vi "PhaseShiftModulation.vi"(0 "PhaseShift":i32, 1 "enable":bool=TRUE, 5 "Period":u32, 7 "Deadband":u8) -> (4 "PrimaryCmds":T1, 6 "SecondaryCmds":T1)   [LabVIEW 2016]
uses:
  BridgeCmds.ctl
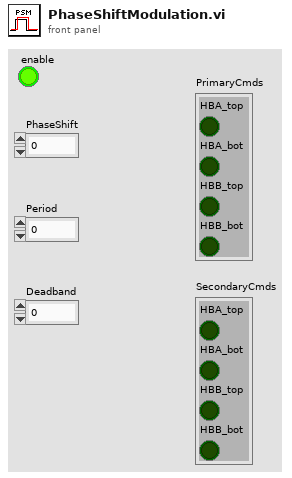
[diagram p1: front panel]
types:
  T1 = typedef "BridgeCmds.ctl" = cluster{"HBA_top":bool, "HBA_bot":bool, "HBB_top":bool, "HBB_bot":bool}
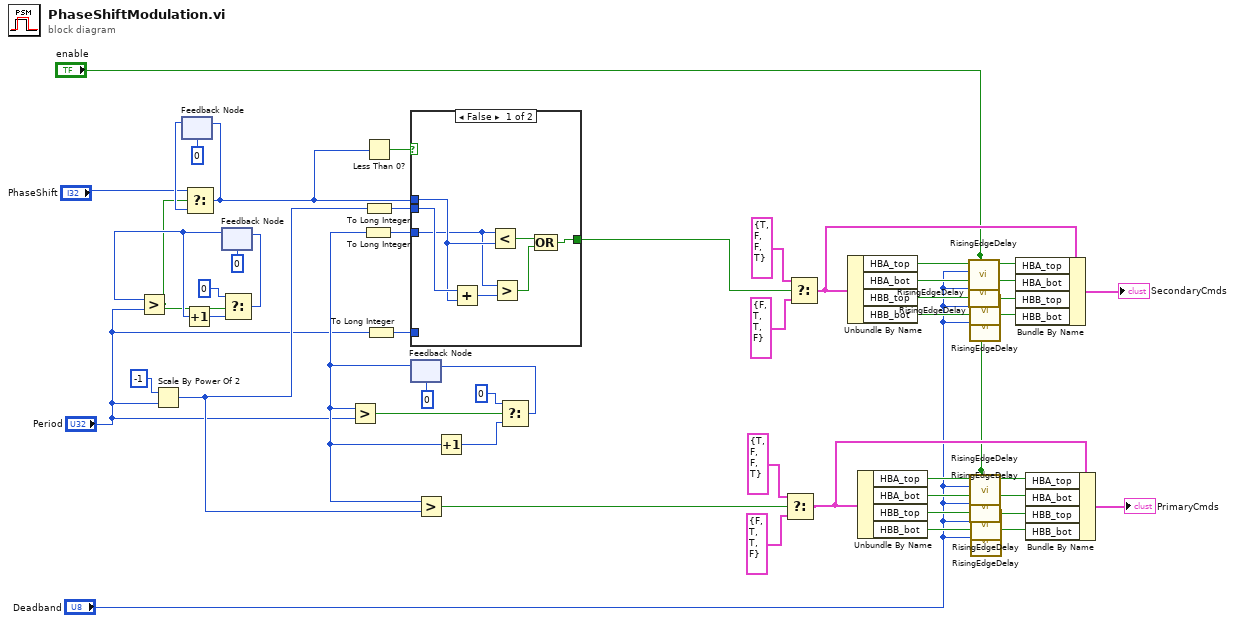
[diagram p0: block diagram]
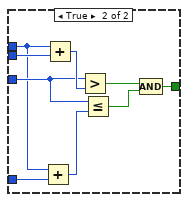
[diagram p2: hidden frame]
diagram:
  n1 = Scale By Power Of 2(n=i16 -1, x="Period") -> (x*2^n=w7:u32)
  n2 = feedback #1(0) -> (w39:i32)
  n3 = feedback #2(u32 0) -> (w41:u32)
  n4 = Greater?(x=w41, y="Period") -> (0:w37:bool)
  n5 = Increment(x=w41) -> (x+1=w43:u32)
  n6 = Select(t="PhaseShift", s=w37, f=w39) -> (s? t:f=w2:i32)
  n7 = feedback-in #1(w2) -> ()
  n8 = Select(t=u32 0, s=w37, f=w43) -> (s? t:f=w42:u32)
  n9 = feedback-in #2(w42) -> ()
  n10 = Less Than 0?(x=w2) -> (x < 0?=w1:bool)
  n11 = To Long Integer(number=w7) -> (32bit integer=w8:i32)
  n12 = To Long Integer(number="Period") -> (32bit integer=w4:i32)
  n13 = feedback #3(u32 0) -> (w6:u32)
  n14 = Greater?(x=w6, y="Period") -> (0:w47:bool)
  n15 = To Long Integer(number=w6) -> (32bit integer=w5:i32)
  n16 = case shown="False" w1 {
    tunnel: [w57 w64] -> w9
    tunnel: w8 -> [w56 w63]
    tunnel: w5 -> [w53 w62]
    tunnel: w4 -> [_ w61]
    tunnel: w2 -> [w55 w59]
    frame False {
      n17 = Add(x=w56, y=w55) -> (x+y=w54:i32)
      n18 = Less?(x=w53, y=w55) -> (x < y?=w58:bool)
      n19 = Greater?(x=w53, y=w54) -> (0:w52:bool)
      n20 = Compound Arithmetic op=OR(w58, w52) -> (w57:bool)
    }
    frame True {
      n21 = Add(x=w59, y=w61) -> (x+y=w60:i32)
      n22 = Add(x=w59, y=w63) -> (x+y=w67:i32)
      n23 = Greater?(x=w62, y=w67) -> (0:w66:bool)
      n24 = Less Or Equal?(x=w62, y=w60) -> (x <= y?=w65:bool)
      n25 = Compound Arithmetic op=AND(w66, w65) -> (w64:bool)
    }
  }
  n26 = Greater?(x=w6, y=w7) -> (0:w10:bool)
  n27 = Increment(x=w6) -> (x+1=w48:u32)
  n28 = Select(t=u32 0, s=w47, f=w48) -> (s? t:f=w46:u32)
  n29 = feedback-in #3(w46) -> ()
  n30 = Select(t=T1 {"HBA_top"=TRUE, "HBA_bot"=FALSE, "HBB_top"=FALSE, "HBB_bot"=TRUE} ("PrimaryCmds"), s=w10, f=T1 {"HBA_top"=FALSE, "HBA_bot"=TRUE, "HBB_top"=TRUE, "HBB_bot"=FALSE} ("PrimaryCmds")) -> (s? t:f=w14:T1)
  n31 = Select(t=T1 {"HBA_top"=TRUE, "HBA_bot"=FALSE, "HBB_top"=FALSE, "HBB_bot"=TRUE} ("PrimaryCmds"), s=w9, f=T1 {"HBA_top"=FALSE, "HBA_bot"=TRUE, "HBB_top"=TRUE, "HBB_bot"=FALSE} ("PrimaryCmds")) -> (s? t:f=w28:T1)
  n32 = Unbundle By Name(w28) -> ("HBA_top"=w32:bool, "HBA_bot"=w31:bool, "HBB_top"=w30:bool, "HBB_bot"=w29:bool)
  n33 = Unbundle By Name(w14) -> ("HBA_top"=w22:bool, "HBA_bot"=w21:bool, "HBB_top"=w20:bool, "HBB_bot"=w19:bool)
  n34 = call "RisingEdgeDelay.vi"("enable?"="enable", "Deadtime (iterations)"="Deadband", "Input"=w32) -> ("Output"=w26:bool)  [unwired: 8 in]
  n35 = call "RisingEdgeDelay.vi"("enable?"="enable", "Deadtime (iterations)"="Deadband", "Input"=w31) -> ("Output"=w25:bool)  [unwired: 8 in]
  n36 = call "RisingEdgeDelay.vi"("enable?"="enable", "Deadtime (iterations)"="Deadband", "Input"=w30) -> ("Output"=w24:bool)  [unwired: 8 in]
  n37 = call "RisingEdgeDelay.vi"("enable?"="enable", "Deadtime (iterations)"="Deadband", "Input"=w29) -> ("Output"=w23:bool)  [unwired: 8 in]
  n38 = call "RisingEdgeDelay.vi"("enable?"="enable", "Deadtime (iterations)"="Deadband", "Input"=w22) -> ("Output"=w18:bool)  [unwired: 8 in]
  n39 = call "RisingEdgeDelay.vi"("enable?"="enable", "Deadtime (iterations)"="Deadband", "Input"=w21) -> ("Output"=w17:bool)  [unwired: 8 in]
  n40 = call "RisingEdgeDelay.vi"("enable?"="enable", "Deadtime (iterations)"="Deadband", "Input"=w20) -> ("Output"=w16:bool)  [unwired: 8 in]
  n41 = call "RisingEdgeDelay.vi"("enable?"="enable", "Deadtime (iterations)"="Deadband", "Input"=w19) -> ("Output"=w15:bool)  [unwired: 8 in]
  n42 = Bundle By Name(cluster=w28, "HBA_top"=w26, "HBA_bot"=w25, "HBB_top"=w24, "HBB_bot"=w23) -> (→"SecondaryCmds":T1)
  n43 = Bundle By Name(cluster=w14, "HBA_top"=w18, "HBA_bot"=w17, "HBB_top"=w16, "HBB_bot"=w15) -> (→"PrimaryCmds":T1)
